vi "Global Visa Ref.vi"() -> ()   [LabVIEW 2016]
panel:
  out "VISA ref":refnum<visa-resource-name>="34970A"
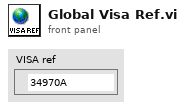
[diagram p1: front panel]
diagram:
